vi "z closure zid call.vi"(8 "error in (no error)":errorcluster, 10 "z_id":cluster{}, 11 "closure":cluster{}) -> (0 "error out":errorcluster)   [LabVIEW 2021, in "zenohc.lvlib"]
doc: "void z_closure_zid_call(const struct z_loaned_closure_zid_t *closure,\n const struct z_id_t *z_id);"
uses:
  zenohc.lvlib
  zenohc.dll
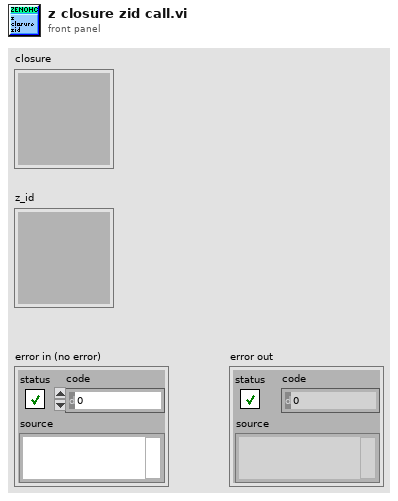
[diagram p1: front panel]
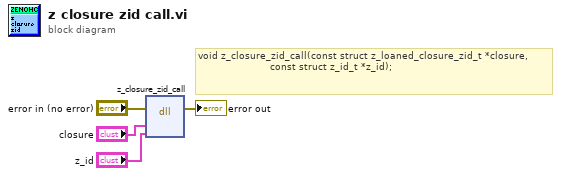
[diagram p0: block diagram]
diagram:
  # "void z_closure_zid_call(const struct z_loaned_closure_zid_t *closure,\n                        const struct z_id_t *z_id);"
  n1 = dll-call lib="D:/dev/zenoh_labview/zenohc/zenohc.*" fn="z_closure_zid_call"(error in="error in (no error)", "closure"="closure", "z_id"="z_id") -> (error out=→"error out":errorcluster)  [unwired: 5 in, 1 out]
